vi "populateTSR.vi"(0 "reference in":refnum<class "excelFile.lvclass">, 1 "TSR_details":T1={"Company/Institution:"="", "Address:"="", "Department:"="", "City:"="", "Post Code:"="", "Country:"="", "Contact:"="", "Ref:"="", "Issue description:"="", "Actions:"="", "TYPE:"="Repair", "Shipping:"=0, "Discount:"=0, "dataIN"=[], "Device type:"="microQuark", "Serial Number:"="", "PMC number:"="", "Labour Hours:"=0.0, "Service Location:"=FALSE, "start_hour"="", "end_hour"=""}, 4 "data":string[][](array[string]), 5 "error in (no error)":errorcluster) -> (14 "reference out":refnum<class "excelFile.lvclass">, 16 "latest_TSR_path":string, 19 "error out":errorcluster)   [LabVIEW 2015, in "excelFile.lvclass"]
uses:
  excelFile.lvclass
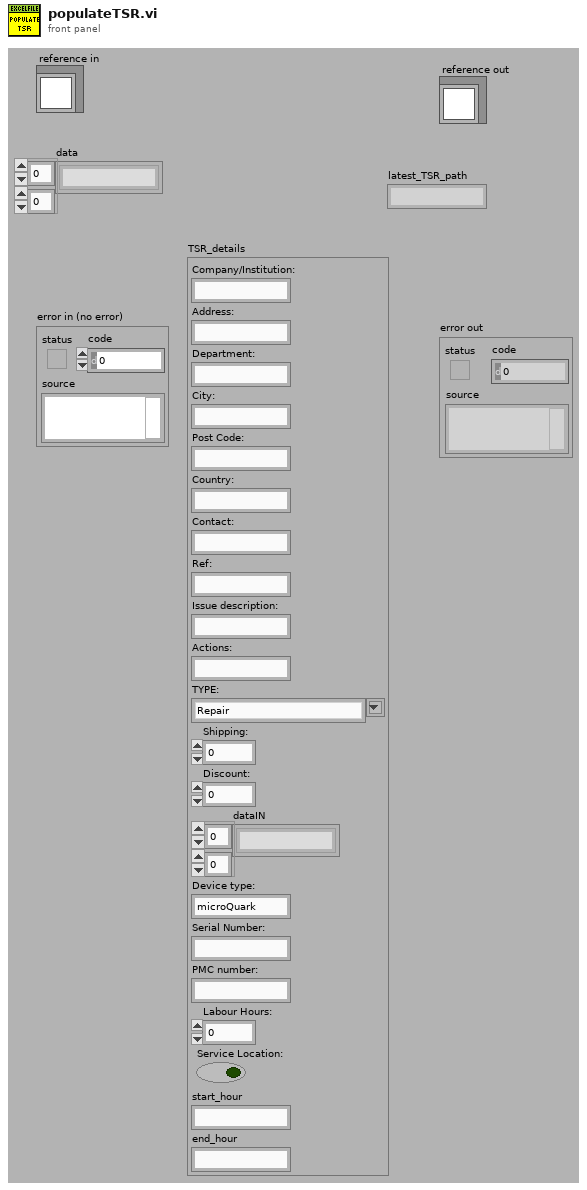
[diagram p1: front panel]
types:
  T1 = cluster{"Company/Institution:":string, "Address:":string, "Department:":string, "City:":string, "Post Code:":string, "Country:":string, "Contact:":string, "Ref:":string, "Issue description:":string, "Actions:":string, "TYPE:":string, "Shipping:":i32, "Discount:":i32, "dataIN":string[][], "Device type:":string, "Serial Number:":string, "PMC number:":string, "Labour Hours:":dbl, "Service Location:":bool, "start_hour":string, "end_hour":string}
  T2 = typedef "excelFile.lvclass/ObjectAttributesRef.ctl" = refnum<data-value>
  T3 = typedef "excelFile.lvclass/ObjectAttributes.ctl" = cluster{"MyAttribute":dbl, "path":string, "Refnum Excel":cluster{"Excel._Application":refnum<k7>, "Workbooks":refnum<k7>, "Open":refnum<k7>}, "data":string[][][], "save":bool, "fileType":T4, "rowsColor":u32[], "python_ref":refnum<class "python.lvclass">, "items_rows":i32[], "excel_range":i32[][], "TSR":cluster{"number":string, "TSR_path":path, "service_path":path, "email_to":string}}
  T4 = typedef "excelFile.lvclass/fileType.ctl" = enum16{"devices", "items", "partsTracking", "TSR"}
  T5 = cluster{"Excel._Application":refnum<k7>, "Workbooks":refnum<k7>, "Open":refnum<k7>}
  T6 = cluster{"number":string, "TSR_path":path, "service_path":path, "email_to":string}
  T7 = cluster{"Excel._Application":refnum<k7>, "Workbooks":refnum<k7>, "Open":refnum<k7>, "Worksheets":refnum<k7>, "Excel._Worksheet":refnum<k7>}
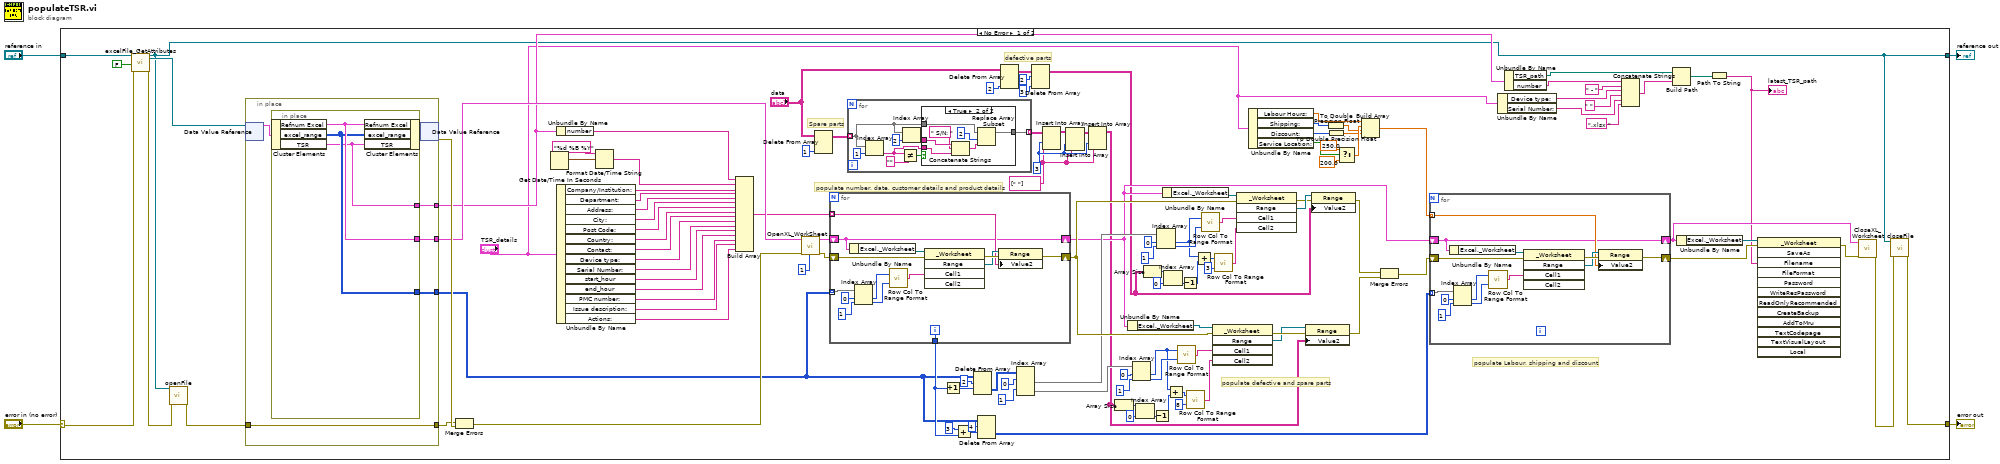
[diagram p0: block diagram]
diagram:
  n1 = case shown="No Error" "error in (no error)" {
    selector: "error in (no error)" -> [w46 w181]
    tunnel: [w59 w181] -> w3
    tunnel: [w11 w180] -> w1
    tunnel: "reference in" -> [w125 w180]
    frame No Error {
      w14 = string[] [" "] ("new element/subarray")
      w15 = 3 ("index")
      # "populate Labour, shipping and discount"
      # "populate defective and spare parts"
      # "defective parts"
      # "Spare parts"
      # "populate number, date, customer details and product details"
      n2 = call "excelFile_GetAttributes.vi"("reference in"=w125, "return data? (T)"=FALSE, "error in (no error)"=w46) -> ("reference out"=w11:refnum<class "excelFile.lvclass">, "attributes ref"=w123:T2, "error out"=w13:errorcluster)  [unwired: 13 in, 1 out]
      n3 = call "openFile.vi"("reference in"=w11, "error in (no error)"=w13) -> ("error out"=w12:errorcluster)  [unwired: 16 in, 1 out]
      n4 = in-place {
        in-place-border: w12 -> [w174]
        in-place-border: [w174] -> w126
        in-place-border: [w173] -> w108
        in-place-border: [w172] -> w8
        in-place-border: [w171] -> w58
        n5 = in-place-dvr #1(w123) -> (w175:T3)  [unwired: 1 out]
        n6 = in-place {
          in-place-border: [w179] -> w173
          in-place-border: [w178] -> w172
          in-place-border: [w177] -> w171
          n7 = in-place-cluster #2(w175) -> ("Refnum Excel"=w179:T5, "excel_range"=w178:i32[][], "TSR"=w177:T6)
          n8 = in-place-cluster #2("Refnum Excel"=w179, "excel_range"=w178, "TSR"=w177) -> (w176:T3)
        }
        n9 = in-place-dvr #1(w176) -> (w127:errorcluster)  [unwired: 1 out]
      }
      n10 = Merge Errors(w126, w127) -> (w47:errorcluster)
      n11 = Get Date/Time In Seconds() -> (seconds since 1Jan1904=w122:timestamp)
      n12 = Unbundle By Name(w58) -> ("number"=w45:string)
      n13 = Unbundle By Name("TSR_details") -> ("Company/Institution:"=w120:string, "Department:"=w119:string, "Address:"=w118:string, "City:"=w117:string, "Post Code:"=w116:string, "Country:"=w115:string, "Contact:"=w114:string, "Device type:"=w113:string, "Serial Number:"=w112:string, "start_hour"=w9:string, "end_hour"=w7:string, "PMC number:"=w111:string, "Issue description:"=w110:string, "Actions:"=w109:string)
      n14 = Format Date/Time String(time format string (%c)="%d %B %Y", seconds (now)=w122) -> (date/time string=w44:string)  [unwired: 1 in]
      n15 = Build Array(w45, w44, w120, w119, w118, w117, w116, w115, w114, w113, w112, w9, w7, w111, w110, w109) -> (w105:string[])
      n16 = call <userlib>:"OpenXL_WorkSheet.vi"("Sheet"=1, "error in (no error)"=w47, "Refnum Cluster In"=w108) -> ("error out"=w106:errorcluster, "Refnum Cluster Out"=w107:T7)  [unwired: 7 in]
      n17 = Delete From Array(array="data", index (col)=1 ("disabled index (col)")) -> (array with subset deleted=w20:string[][])  [unwired: 2 in, 1 out]
      n18 = for {
        shift-right: [w159] -> w80
        shift-left: w106 -> [w161]
        shift-right: [w158] -> w66
        shift-left: w107 -> [w158]
        tunnel: w8 -> [w166] mode=indexing
        tunnel: w105 -> [w160] mode=indexing
        tunnel: [w157] -> w74
        i -> [w157]
        n19 = Unbundle By Name(w158) -> ("Excel._Worksheet"=w167:refnum<k7>)
        n20 = Index Array(array=w166, index #1=0 ("index"), index #2=1 ("index")) -> (element #1=w163:i32, element #2=w162:i32)
        n21 = call <userlib>:"Row Col To Range Format.vi"("Column"=w162, "Row"=w163) -> ("Output String"=w170:string)
        n22 = invoke class="_Worksheet" method="Range"(reference=w167, error in=w161, "Cell1"=w170) -> (error out=w169:errorcluster, "Range"=w168:refnum<k7>)  [unwired: 2 in, 3 out]
        n23 = property class="Range"(reference=w168, error in=w169, "Value2"=w160) -> (error out=w159:errorcluster)  [unwired: 1 out]
      }
      n24 = for {
        tunnel: w20 -> [w132] mode=indexing
        tunnel: [w129] -> w19 mode=indexing
        n25 = Index Array(array=w132, index=1) -> (element=w128:string)
        n26 = Not Equal?(x=w128, y="") -> (x != y?=w133:bool)
        n27 = Index Array(array=w132, index=2) -> (element=w130:string)
        n28 = case shown="True" w133 {
          tunnel: w132 -> [w136 w143]
          tunnel: w130 -> [_ w140]
          tunnel: [w136 w141] -> w129
          tunnel: w128 -> [_ w137]
          frame False {
          }
          frame True {
            n29 = Concatenate Strings(w140, " S/N: " ("string"), w137) -> (w139:string)
            n30 = Replace Array Subset(array=w143, new element=w139, index=2) -> (w141:string[])
          }
        }
      }
      n31 = Increment(x=w74) -> (x+1=w91:i32)
      n32 = Add(x=3, y=w74) -> (x+y=w75:i32)
      n33 = Delete From Array(array=w8, length=2 ("index"), index (row)=w91) -> (deleted portion=w43:i32[][])  [unwired: 1 in, 1 out]
      n34 = Delete From Array(array=w8, length=4 ("index"), index (row)=w75) -> (deleted portion=w42:i32[][])  [unwired: 1 in, 1 out]
      n35 = Delete From Array(array="data", index (col)=2 ("disabled index (col)")) -> (array with subset deleted=w101:string[][])  [unwired: 2 in, 1 out]
      n36 = Index Array(array=w43, index (row) #1=0 ("index"), index (row) #2=1 ("index")) -> (element #1=w78:i32[], element #2=w79:i32[])  [unwired: 2 in]
      n37 = Delete From Array(array=w101, length=2 ("disabled index (col)"), index (col)=3 ("disabled index (col)")) -> (array with subset deleted=w37:string[][])  [unwired: 1 in, 1 out]
      n38 = Insert Into Array(array=w19, index (col)=w15, new element=w14) -> (w18:string[][])  [unwired: 1 in]
      n39 = Insert Into Array(array=w18, index (col)=w15, new element=w14) -> (w17:string[][])  [unwired: 1 in]
      n40 = Insert Into Array(array=w17, index (col)=w15, new element=w14) -> (w16:string[][])  [unwired: 1 in]
      n41 = Array Size(array=w16) -> (size(s)=w32:i32[])
      n42 = Unbundle By Name(w66) -> ("Excel._Worksheet"=w94:refnum<k7>)
      n43 = Index Array(array=w79, index #1=0 ("index"), index #2=1 ("index")) -> (element #1=w26:i32, element #2=w88:i32)
      n44 = Index Array(array=w32, index=0) -> (element=w28:i32)
      n45 = Array Size(array=w37) -> (size(s)=w36:i32[])
      n46 = Decrement(x=w28) -> (x-1=w22:i32)
      n47 = Index Array(array=w78, index #1=0 ("index"), index #2=1 ("index")) -> (element #1=w23:i32, element #2=w87:i32)
      n48 = Unbundle By Name(w66) -> ("Excel._Worksheet"=w84:refnum<k7>)
      n49 = Index Array(array=w36, index=0) -> (element=w25:i32)
      n50 = Add(x=w26, y=w22) -> (x+y=w27:i32)
      n51 = call <userlib>:"Row Col To Range Format.vi"("Column"=w88, "Row"=w26) -> ("Output String"=w97:string)
      n52 = Decrement(x=w25) -> (x-1=w21:i32)
      n53 = call <userlib>:"Row Col To Range Format.vi"("Column"=8, "Row"=w27) -> ("Output String"=w29:string)
      n54 = Add(x=w23, y=w21) -> (x+y=w24:i32)
      n55 = call <userlib>:"Row Col To Range Format.vi"("Column"=w87, "Row"=w23) -> ("Output String"=w81:string)
      n56 = invoke class="_Worksheet" method="Range"(reference=w94, error in=w80, "Cell1"=w97, "Cell2"=w29) -> (error out=w96:errorcluster, "Range"=w95:refnum<k7>)  [unwired: 1 in, 3 out]
      n57 = call <userlib>:"Row Col To Range Format.vi"("Column"=3, "Row"=w24) -> ("Output String"=w34:string)
      n58 = invoke class="_Worksheet" method="Range"(reference=w84, error in=w80, "Cell1"=w81, "Cell2"=w34) -> (error out=w82:errorcluster, "Range"=w83:refnum<k7>)  [unwired: 1 in, 3 out]
      n59 = Unbundle By Name("TSR_details") -> ("Labour Hours:"=w72:dbl, "Shipping:"=w39:i32, "Discount:"=w41:i32, "Service Location:"=w71:bool)
      n60 = property class="Range"(reference=w95, error in=w96, "Value2"=w16) -> (error out=w76:errorcluster)  [unwired: 1 out]
      n61 = property class="Range"(reference=w83, error in=w82, "Value2"=w37) -> (error out=w77:errorcluster)  [unwired: 1 out]
      n62 = To Double Precision Float(number=w39) -> (double precision float=w6:dbl)
      n63 = To Double Precision Float(number=w41) -> (double precision float=w5:dbl)
      n64 = Select(t=250.0, s=w71, f=200.0) -> (s? t:f=w40:dbl)
      n65 = Build Array(w72, w40, w6, w5) -> (w68:dbl[])
      n66 = Merge Errors(w77, w76) -> (w67:errorcluster)
      n67 = for {
        shift-right: [w145] -> w63
        shift-left: w67 -> [w147]
        shift-right: [w144] -> w62
        shift-left: w66 -> [w144]
        tunnel: w42 -> [w152] mode=indexing
        tunnel: w68 -> [w146] mode=indexing
        n68 = Unbundle By Name(w144) -> ("Excel._Worksheet"=w153:refnum<k7>)
        n69 = Index Array(array=w152, index #1=0 ("index"), index #2=1 ("index")) -> (element #1=w149:i32, element #2=w148:i32)
        n70 = call <userlib>:"Row Col To Range Format.vi"("Column"=w148, "Row"=w149) -> ("Output String"=w156:string)
        n71 = invoke class="_Worksheet" method="Range"(reference=w153, error in=w147, "Cell1"=w156) -> (error out=w155:errorcluster, "Range"=w154:refnum<k7>)  [unwired: 2 in, 3 out]
        n72 = property class="Range"(reference=w154, error in=w155, "Value2"=w146) -> (error out=w145:errorcluster)  [unwired: 1 out]
      }
      n73 = Unbundle By Name("TSR_details") -> ("Device type:"=w55:string, "Serial Number:"=w53:string)
      n74 = Unbundle By Name(w58) -> ("TSR_path"=w51:path, "number"=w57:string)
      n75 = Concatenate Strings(w57, " - ", w55, " ", w53, ".xlsx ") -> (w50:string)
      n76 = Build Path(base path=w51, name or relative path=w50) -> (appended path=w49:path)
      n77 = Unbundle By Name(w62) -> ("Excel._Worksheet"=w64:refnum<k7>)
      n78 = Path To String(path=w49) -> (string=w48:string)
      "latest_TSR_path" <- w48
      n79 = invoke class="_Worksheet" method="SaveAs"(reference=w64, error in=w63, "Filename"=w48) -> (error out=w61:errorcluster)  [unwired: 10 in, 12 out]
      n80 = call <userlib>:"CloseXL_Worksheet.vi"("error in (no error)"=w61, "Refnum Cluster In"=w62) -> ("error out"=w60:errorcluster)  [unwired: 8 in, 1 out]
      n81 = call "closeFile.vi"("error in (no error)"=w60, "reference in"=w11) -> ("error out"=w59:errorcluster)  [unwired: 8 in, 1 out]
    }
    frame Error {
    }
  }
  "error out" <- w3
  "reference out" <- w1
